vi "Mask the Password.vi"(8 "error in (no error)":errorcluster, 10 "Cmd String in":string) -> (0 "error out":errorcluster, 2 "Cmd String out":string)   [LabVIEW 2017, in "FTP.lvlib" / "FTP.lvclass"]
uses:
  FTP.lvclass
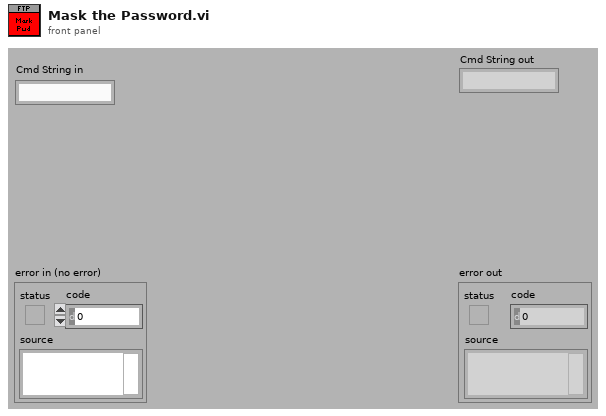
[diagram p1: front panel]
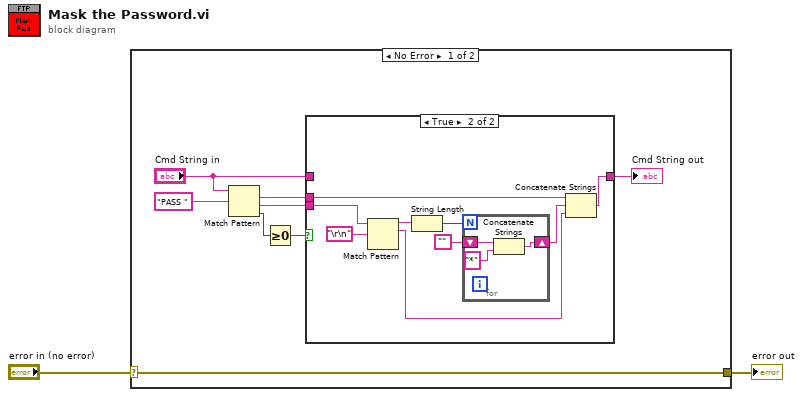
[diagram p0: block diagram]
diagram:
  n1 = case shown="No Error" "error in (no error)" {
    selector: "error in (no error)" -> [w10 w24]
    tunnel: [w10 w24] -> w1
    frame No Error {
      n2 = Match Pattern(string="Cmd String in", regular expression="PASS ") -> (match substring=w3:string, after substring=w6:string, offset past match=w7:i32)  [unwired: 1 in, 1 out]
      n3 = Greater Or Equal To 0?(x=w7) -> (x >= 0?=w8:bool)
      n4 = case shown="True" w8 {
        tunnel: "Cmd String in" -> [w11 _]
        tunnel: [w11 w17] -> w4
        tunnel: w6 -> [_ w15]
        tunnel: w3 -> [_ w16]
        frame False {
        }
        frame True {
          n5 = Match Pattern(string=w15, regular expression="\r\n") -> (before substring=w14:string, match substring=w12:string)  [unwired: 1 in, 2 out]
          n6 = String Length(string=w14) -> (length=w20:i32)
          n7 = for {
            N: w20 -> [_]
            shift-right: [w21] -> w18
            shift-left: "" -> [w23]
            n8 = Concatenate Strings(w23, "*") -> (w21:string)
          }
          n9 = Concatenate Strings(w16, w18, w12) -> (w17:string)
        }
      }
      "Cmd String out" <- w4
    }
    frame Error {
    }
  }
  "error out" <- w1
